vi "Robot Information.vi"   [LabVIEW 2018]
uses:
  Robot Information Global.vi
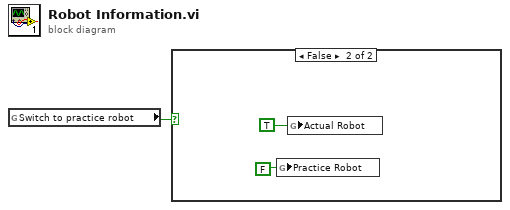
[diagram p0: block diagram]
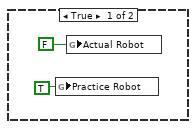
[diagram p2: hidden frame]
diagram:
  n1 = global read "Robot Information Global.vi" "Switch to practice robot"() -> (w1:bool)
  n2 = case shown="False" w1 {
    frame True {
      n3 = global write "Robot Information Global.vi" "Practice Robot"(TRUE) -> ()
      n4 = global write "Robot Information Global.vi" "Actual Robot"(FALSE ("Practice Robot")) -> ()
    }
    frame False {
      n5 = global write "Robot Information Global.vi" "Practice Robot"(FALSE) -> ()
      n6 = global write "Robot Information Global.vi" "Actual Robot"(TRUE ("Practice Robot")) -> ()
    }
  }
